vi "Check Point Inside.vi"(10 "rect":T2, 11 "Point In":cluster{"x":T1, "y":T1}) -> (2 "Inside":bool, 3 "Point":cluster{"x":T1, "y":T1})   [LabVIEW 2020, in "FlexBlock.xnode"]
uses:
  FlexBlock.xnode
  <vilib>/XNodeSupport/XNodeInt.ctl
  <vilib>/XNodeSupport/NI_XNodeSupport.lvlib
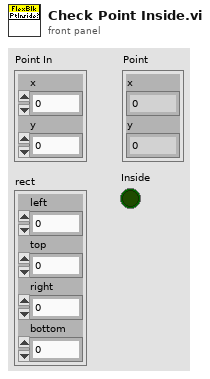
[diagram p1: front panel]
types:
  T1 = typedef "NI_XNodeSupport.lvlib/XNodeInt.ctl" = i32
  T2 = cluster{"left":i16, "top":i16, "right":i16, "bottom":i16}
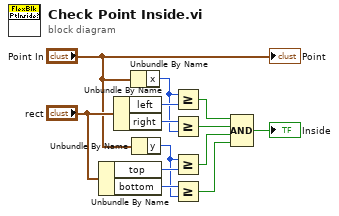
[diagram p0: block diagram]
diagram:
  n1 = Unbundle By Name("rect") -> ("top"=w12:i16, "bottom"=w11:i16)
  n2 = Unbundle By Name("rect") -> ("left"=w9:i16, "right"=w8:i16)
  n3 = Unbundle By Name("Point In") -> ("x"=w6:T1)
  n4 = Unbundle By Name("Point In") -> ("y"=w10:T1)
  n5 = Greater Or Equal?(x=w6, y=w9) -> (x >= y?=w5:bool)
  n6 = Greater Or Equal?(x=w8, y=w6) -> (x >= y?=w4:bool)
  n7 = Greater Or Equal?(x=w10, y=w12) -> (x >= y?=w3:bool)
  n8 = Greater Or Equal?(x=w11, y=w10) -> (x >= y?=w2:bool)
  n9 = Compound Arithmetic op=AND(w5, w4, w3, w2) -> (→"Inside":bool)
  "Point" <- "Point In"
